vi "题目8.vi"() -> ()   [LabVIEW 2017]
panel:
  out "y":dbl
  in  "n":dbl
  in  "m":dbl
  in  "x":dbl
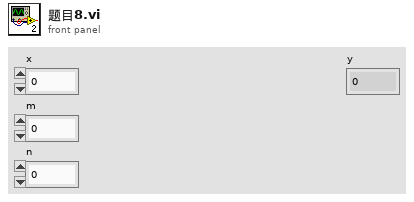
[diagram p1: front panel]
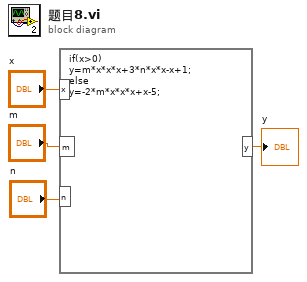
[diagram p0: block diagram]
diagram:
  n1 = formula code="if(x>0)\ny=m*x*x*x+3*n*x*x-x+1;\nelse\ny=-2*m*x*x*x+x-5;"("x"="x", "m"="m", "n"="n") -> ("y"=→"y":dbl)
